vi "Configure.vi"(6 "Input channel":i32, 8 "error in":errorcluster, 9 "Digital capture samples":u32, 10 "Digital capture sample rate":dbl, 11 "gRPC session in":T1) -> (0 "error out":errorcluster, 3 "gRPC session out":T1)   [LabVIEW 2021, in "dcvmDPI_AD7606B_clientImpl.lvlib"]
uses:
  dcvmDPI_AD7606B_clientImpl.lvlib
  <vilib>/gRPC/LabVIEW gRPC Library/Shared/grpcId.ctl
  dcvmDPI_AD7606B_client/RPC Messages/dcvmDPI_ConfigureRequest.ctl
  dcvmDPI_AD7606B_client/dcvmDPI_AD7606B_client.lvlib
  <vilib>/gRPC/LabVIEW gRPC Library/grpc-lvsupport-release.lvlib
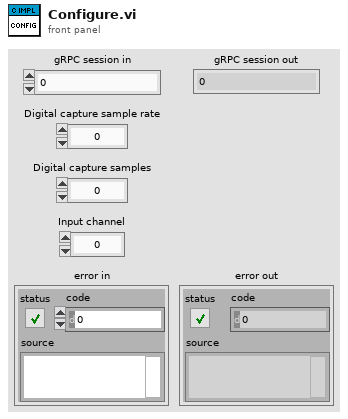
[diagram p1: front panel]
types:
  T1 = typedef "grpc-lvsupport-release.lvlib/grpcId.ctl" = u64
  T2 = typedef "dcvmDPI_AD7606B_client.lvlib/dcvmDPI_ConfigureRequest.ctl" = cluster{"digital_capture_samples":u32, "digital_capture_sample_rate":dbl, "input_channel":i32}
  T3 = typedef "dcvmDPI_AD7606B_client.lvlib/dcvmDPI_ConfigureResponse.ctl" = cluster{"error":T4}
  T4 = typedef "dcvmDPI_AD7606B_client.lvlib/dcvmDPI_ErrorResponse.ctl" = cluster{"error_number":i32, "error_description":string}
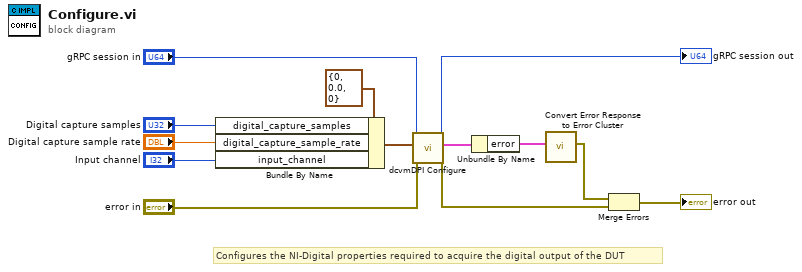
[diagram p0: block diagram]
diagram:
  # "Configures the NI-Digital properties required to acquire the digital output of the DUT"
  n1 = Bundle By Name(cluster=T2 {"digital_capture_samples"=0, "digital_capture_sample_rate"=0.0, "input_channel"=0} ("Request Data"), "digital_capture_samples"="Digital capture samples", "digital_capture_sample_rate"="Digital capture sample rate", "input_channel"="Input channel") -> (w10:T2)
  n2 = call "dcvmDPI Configure.vi"("error in"="error in", "Request Data"=w10, "gRPC ID"="gRPC session in") -> ("error out"=w2:errorcluster, "Response Data"=w5:T3, "gRPC ID out"=→"gRPC session out":T1)  [unwired: 6 in]
  n3 = Unbundle By Name(w5) -> ("error"=w4:T4)
  n4 = call "Convert Error Response to Error Cluster.vi"("Error response"=w4) -> ("error out"=w3:errorcluster)  [unwired: 10 in]
  n5 = Merge Errors(w3, w2) -> (→"error out":errorcluster)
